vi "ERR Build Error Item Matrix.vi"(0 "Start Path (Empty:Top Level)":path, 11 "Error In (No Error)":errorcluster) -> (4 "Error Item Matrix":string[][](array[string])=[["TES CFG", "Configuration"], ["TES CTL", "Control Station"], ["TES HSC", "Head Stack Control"], ["TES IT", "Information Transfer"], ["EXP", "Test Executor"], ["TES TEX", "Test Executor"], ["ET REG", "Controls Registry"], ["ET REG IO", "Controls Registry"], ["DIOCOMM", "MAC_DIO Communication"], ["TES TST ABR", "Abrasivity"], ["TES TST BRW", "Basic Read Write"], ["TES TST BSNR", "Broadband SNR"], ["TES TST HCO", "Head Current Optimization"], ["TES TST LRW", "Locate Rewind"], ["TES TST MPMA", "Missing Pulse"], ["TES TST SVA", "Servo Amplitude"], ["TES TST SC", "Servo Capture"], ["TES TST SA", "Signal Amplitude"], ["TES TST SOV", "Signal Overwrite"], ["TES TST SRE", "Signal Resolution"], ["TES TST SSNR", "Skirt SNR"], ["TES TST WVC", "Width Var and Curvature"], ["AG_3325x PRIV", "AG_Clock Generator"], ["AG_3325x PUB", "AG_Clock Generator"], ["AR_HSP PRIV", "AR_Head Stack Positioner"], ["AR_HSP PUB", "AR_Head Stack Positioner"], ["CMRD PRIV", "BT_CM Reader"], ["CMRD PUB", "BT_CM Reader"], ["FL_PM5193 PRIV", "FLK_Clock Generator"], ["FL_PM5193 PUB", "FLK_Clock Generator"], ["HP_81110 PRIV", "HP_Pattern Generator"], ["HP_81110 PUB", "HP_Pattern Generator"], ["HP_SP AN PRIV", "HP_Spectrum Analyzer"], ["HP_SP AN PUB", "HP_Spectrum Analyzer"], ["LC_SCOPE PRIV", "LC_Oscilloscope"], ["LC_SCOPE PUB", "LC_Oscilloscope"], ["LC_SCOPE PUB EXP", "LC_Oscilloscope"], ["MAC_CLK PUB", "MAC_Clock Generator"], ["MAC_LPOS PRIV", "MAC_LPOS"], ["MAC_LPOS PUB", "MAC_LPOS"], ["MAC_MPMA PRIV", "MAC_MPMA"], ["MAC_MPMA PUB 1B", "MAC_MPMA"], ["MAC_MPMA PUB", "MAC_MPMA"], ["MAC_MUX PRIV", "MAC_Multiplexer"], ["MAC_MUX PUB", "MAC_Multiplexer"], ["MAC_RMS PUB", "MAC_RMS Meter"], ["SFTES DAQ PRIV", "MAC_SFTES DAQ"], ["SFTES DAQ PUB", "MAC_SFTES DAQ"], ["MAC_TES PRIV", "MAC_Tape Edge Sensors"], ["MAC_TES PUB", "MAC_Tape Edge Sensors"], ["MAC_TSPT PRIV", "MAC_Transport"], ["MAC_TSPT PUB", "MAC_Transport"], ["MAC_TSPT EOT PRIV", "MAC_Transport EOT"], ["MAC_TSPT EOT PUB", "MAC_Transport EOT"], ["MAC_TSPT IO PRIV", "MAC_Transport IO Controller"], ["MAC_TSPT IO PUB", "MAC_Transport IO Controller"], ["MAC_TSPT DAQ PRIV", "MAC_TSPT DAQ"], ["MAC_TSPT DAQ PUB", "MAC_TSPT DAQ"], ["MAC_WVCMU PRIV", "MAC_WVCMU"], ["MAC_WVCMU PUB", "MAC_WVCMU"], ["MAC_WVCMU PUB DAQ", "MAC_WVCMU"], ["MT_TSPT PRIV", "MT_Transport"], ["MT_TSPT PUB", "MT_Transport"], ["NA_MVP1 PRIV", "NA_MVP1 Positioner"], ["NA_MVP1 PUB", "NA_MVP1 Positioner"], ["PS_RMC PRIV", "PS_Motor Controller"], ["PS_RMC PUB", "PS_Motor Controller"], ["RC_RMS MTR PRIV", "RC_RMS Meter"], ["RC_RMS MTR PUB", "RC_RMS Meter"], ["RS_RMS MTR PRIV", "RS_RMS Meter"], ["RS_RMS MTR PUB", "RS_RMS Meter"], ["VASL_HUM SNS PRIV", "VASL_Humidity Sensor"], ["VASL_HUM SNS PUB", "VASL_Humidity Sensor"]], 15 "Error Out":errorcluster)   [LabVIEW 2011]
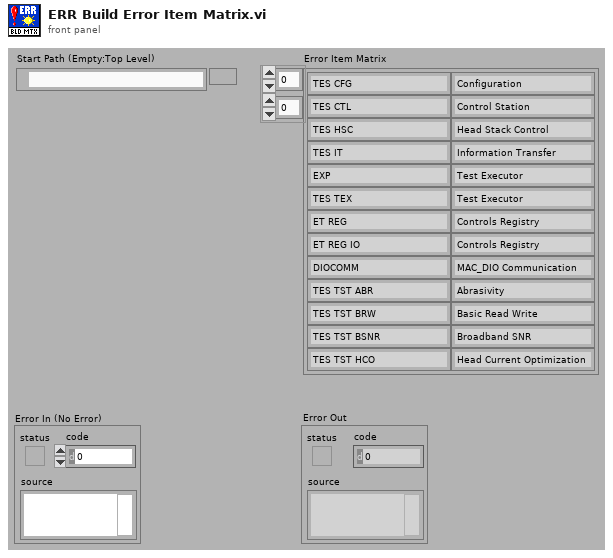
[diagram p1: front panel]
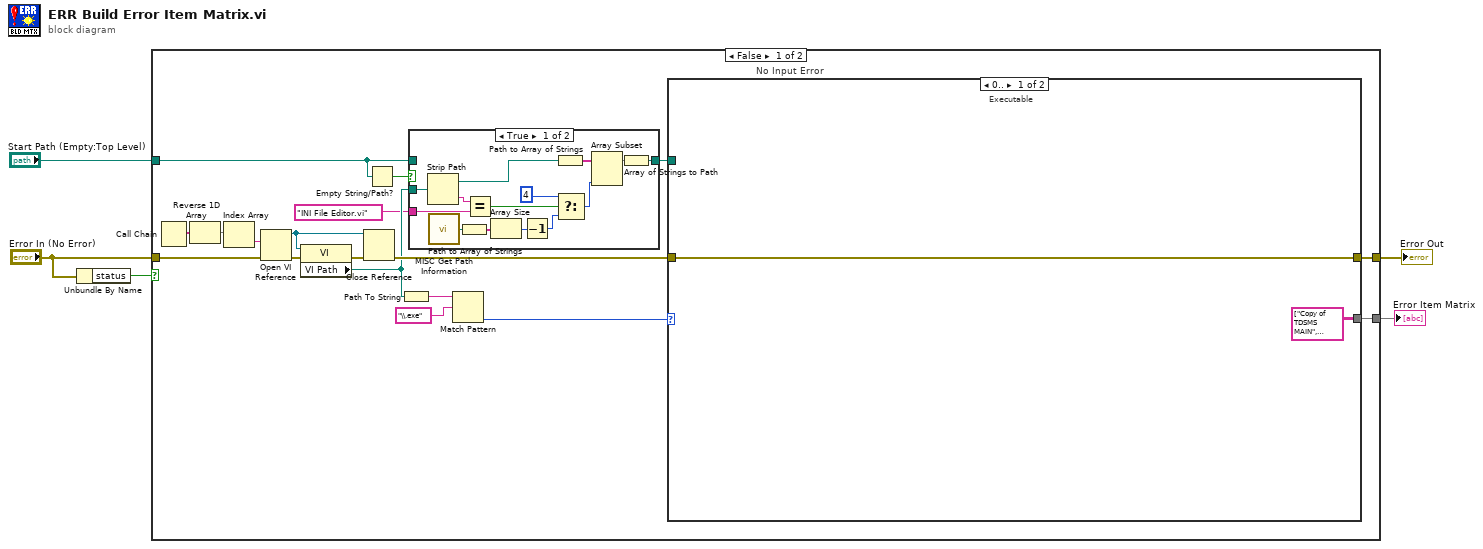
[diagram p0: block diagram]
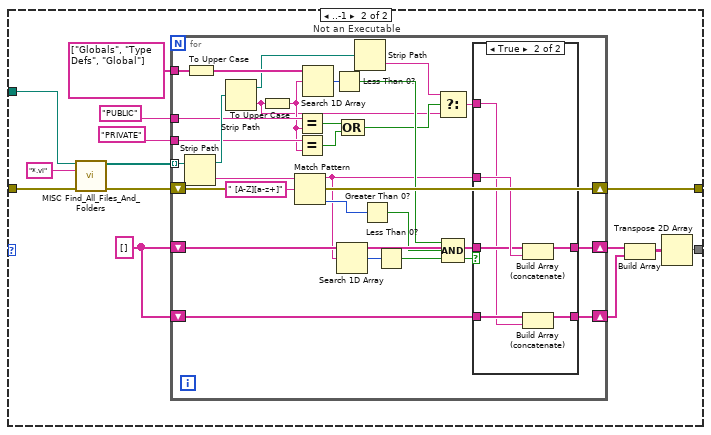
[diagram p2: hidden frame]
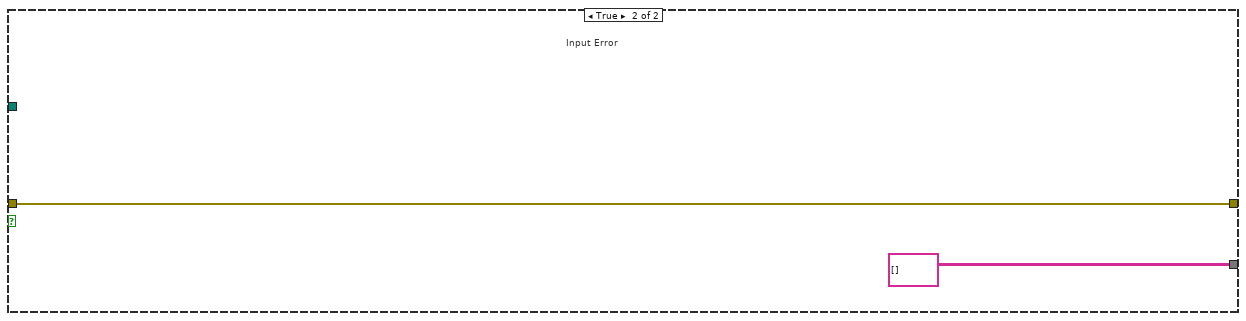
[diagram p5: hidden frame]
diagram:
  n1 = Unbundle By Name("Error In (No Error)") -> ("status"=w2:bool)
  n2 = case shown="False" w2 {
    tunnel: "Start Path (Empty:Top Level)" -> [w21 _]
    tunnel: [w23 w93] -> w4
    tunnel: [w22 string[][] []] -> w1
    tunnel: "Error In (No Error)" -> [w10 w93]
    frame False {
      # "No Input Error"
      n3 = Call Chain() -> (call chain=w11:string[])
      n4 = Reverse 1D Array(array=w11) -> (reversed array=w12:string[])
      n5 = Index Array(array=w12) -> (element=w16:string)  [unwired: 1 in]
      n6 = Open VI Reference(vi path=w16, error in (no error)=w10) -> (vi reference=w15:refnum<vi>, error out=w13:errorcluster)  [unwired: 4 out]
      n7 = property class="VI"(reference=w15, error in=w13) -> (error out=w14:errorcluster, "VI Path"=w8:path)  [unwired: 1 out]
      n8 = Close Reference(reference=w15, error in (no error)=w14) -> (error out=w9:errorcluster)
      n9 = Empty String/Path?(string/path=w21) -> (empty?=w20:bool)
      n10 = Path To String(path=w8) -> (string=w17:string)
      n11 = case shown="True" w20 {
        tunnel: [w88 w91] -> w18
        tunnel: w21 -> [_ w91]
        tunnel: w8 -> [w82 _]
        tunnel: "INI File Editor.vi" ("name") -> [w86 _]
        frame True {
          n12 = Strip Path(path=w82) -> (stripped path=w81:path, name=w87:string)
          n13 = call "MISC Get Path Information.vi"() -> ("Support Directory"=w80:path)  [unwired: 1 in, 14 out]
          n14 = Path to Array of Strings(0:w80) -> (2:w79:string[])  [unwired: 1 out]
          n15 = Equal?(x=w87, y=w86) -> (x = y?=w84:bool)
          n16 = Array Size(array=w79) -> (size(s)=w78:i32)
          n17 = Decrement(x=w78) -> (x-1=w77:i32)
          n18 = Path to Array of Strings(0:w81) -> (2:w90:string[])  [unwired: 1 out]
          n19 = Select(t=4, s=w84, f=w77) -> (s? t:f=w85:i32)
          n20 = Array Subset(array=w90, length=w85) -> (w89:string[])  [unwired: 1 in]
          n21 = Array of Strings to Path(0:w89) -> (2:w88:path)  [unwired: 1 out]
        }
        frame False {
        }
      }
      n22 = Match Pattern(string=w17, regular expression="\\.exe") -> (offset past match=w7:i32)  [unwired: 4 out]
      n23 = case shown="0.." w7 {
        tunnel: [w25 w35] -> w23
        tunnel: [string[][] [["Copy of TDSMS MAIN", "Main"], ["TDSMS MAIN", "Main"], ["TDSMS MAIN TWV", "Main"], ["TDSMS", "Super"], ["ET REG IO", "Controls Registry"], ["Initialize", "Serdrv.llb"], ["Read", "Serdrv.llb"], ["Read until", "Serdrv.llb"], ["Write to", "Serdrv.llb"], ["Add", "Utility.llb"], ["Archive", "Utility.llb"], ["Binary", "Utility.llb"], ["Calculate", "Utility.llb"], ["Convert", "Utility.llb"], ["Error and", "Utility.llb"], ["Error", "Utility.llb"], ["Find and", "Utility.llb"], ["Increment", "Utility.llb"], ["Log", "Utility.llb"], ["Open", "Utility.llb"], ["Open_Create_Replace", "Utility.llb"], ["Read_Write ini", "Utility.llb"], ["Revolution", "Utility.llb"], ["String_Array", "Utility.llb"], ["Wait", "Utility.llb"], ["WMC", "Utility.llb"], ["Write", "Utility.llb"], ["DP41-S PRIV", "DP41-S Strain"], ["DP41-S PUB", "DP41-S Strain"], ["Laser PRIV", "LSM-6100 Laser"], ["Laser PUB", "LSM-6100 Laser"], ["Main PRIV", "Main"], ["Main PUB", "Main"], ["NA_MVP1 PRIV", "NA_MVP1 Positioner"], ["NA_MVP1 PUB", "NA_MVP1 Positioner"], ["TDSMS PRIV", "TDSMS"], ["TDSMS PUB", "TDSMS"], ["VASL_HUM SNS PRIV", "VASL_Humidity Sensor"], ["VASL_HUM SNS PUB", "VASL_Humidity Sensor"]] ("Error Item Matrix") w30] -> w22
        tunnel: w9 -> [w25 w29]
        tunnel: w18 -> [_ w28]
        frame 0.. {
          # "Executable"
        }
        frame ..-1 {
          w36 = string[] []
          # "Not an Executable"
          n24 = call "MISC Find_All_Files_And_Folders.vi"("High Level Directory"=w28, "pattern (*.*)"="*.vi", "error in (no error)"=w29) -> ("All File Paths"=w39:path[], "error out"=w37:errorcluster)  [unwired: 11 out]
          n25 = for {
            tunnel: w39 -> [w68] mode=indexing
            shift-right: [w62] -> w35
            shift-left: w37 -> [w62]
            shift-right: [w63] -> w34
            shift-left: w36 -> [w64]
            shift-right: [w51] -> w33
            shift-left: w36 -> [w61]
            tunnel: string[] ["Globals", "Type Defs", "Global"] -> [w60]
            tunnel: "PUBLIC" -> [w50]
            tunnel: "PRIVATE" -> [w49]
            n26 = Strip Path(path=w68) -> (stripped path=w65:path, name=w67:string)
            n27 = To Upper Case(1:w60) -> (0:w59:string[])
            n28 = Strip Path(path=w65) -> (stripped path=w44:path, name=w41:string)
            n29 = To Upper Case(1:w41) -> (0:w47:string)
            n30 = Match Pattern(string=w67, regular expression=" [A-Z][a-z+]") -> (before substring=w48:string, offset past match=w57:i32)  [unwired: 3 out]
            n31 = Equal?(x=w50, y=w47) -> (x = y?=w46:bool)
            n32 = Equal?(x=w49, y=w47) -> (x = y?=w45:bool)
            n33 = Search 1D Array(1D array=w59, element=w47) -> (index of element=w58:i32)  [unwired: 1 out]
            n34 = Less Than 0?(x=w58) -> (x < 0?=w55:bool)
            n35 = Search 1D Array(1D array=w64, element=w48) -> (index of element=w56:i32)  [unwired: 1 out]
            n36 = Compound Arithmetic op=OR(w46, w45) -> (w43:bool)
            n37 = Strip Path(path=w44) -> (name=w42:string)  [unwired: 1 out]
            n38 = Greater Than 0?(x=w57) -> (x > 0?=w54:bool)
            n39 = Less Than 0?(x=w56) -> (x < 0?=w53:bool)
            n40 = Select(t=w42, s=w43, f=w41) -> (s? t:f=w40:string)
            n41 = Compound Arithmetic op=AND(w55, w54, w53) -> (w52:bool)
            n42 = case shown="True" w52 {
              tunnel: w48 -> [_ w76]
              tunnel: w64 -> [w70 w75]
              tunnel: [w70 w74] -> w63
              tunnel: w61 -> [w69 w73]
              tunnel: [w69 w72] -> w51
              tunnel: w40 -> [_ w71]
              frame False {
              }
              frame True {
                n43 = Build Array (concatenate)(w75, w76) -> (w74:string[])
                n44 = Build Array (concatenate)(w73, w71) -> (w72:string[])
              }
            }
          }
          n45 = Build Array(w34, w33) -> (w32:string[][])
          n46 = Transpose 2D Array(2D array=w32) -> (transposed array=w30:string[][])
        }
      }
    }
    frame True {
      # "Input Error"
    }
  }
  "Error Item Matrix" <- w1
  "Error Out" <- w4
